vi "dfd_Cascaded SOS Form I Transposed Normalization.vi"(7 "scale type":T1, 9 "coefficients b":dbl[](array[numeric]) format="%.2f", 10 "coefficients a":dbl[](array[numeric]) format="%.2f", 11 "x":dbl[](array[numeric])) -> (2 "norm":dbl[](array[numeric]) format="%.2f", 3 "y":dbl[](array[numeric]))   [LabVIEW 2017, in "NI_DigFilter_FXP.lvlib"]
uses:
  <vilib>/addons/Digital Filter Design/NI_DigFilter_FXP.lvlib
  <vilib>/addons/Digital Filter Design/_Objects.llb/DFD Coef Norm Type.ctl
  <vilib>/addons/Digital Filter Design/NI_DigFilterLicensed.lvlib
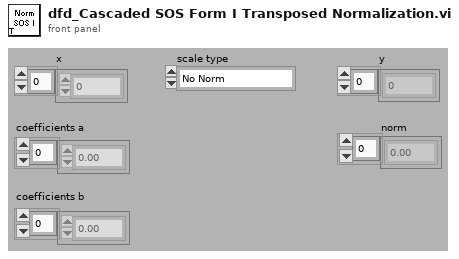
[diagram p1: front panel]
types:
  T1 = typedef "NI_DigFilterLicensed.lvlib/DFD Coef Norm Type.ctl" = enum16{"No Norm", "Time Domain 1-Norm", "Time Domain 2-Norm", "Time Domain Inf-Norm"}
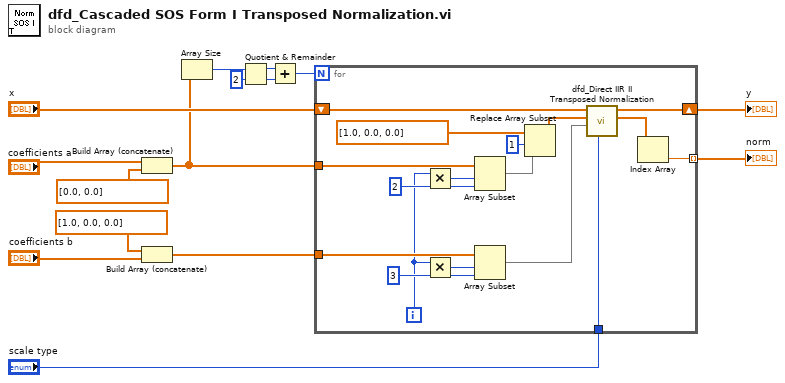
[diagram p0: block diagram]
diagram:
  n1 = Build Array (concatenate)("coefficients a", dbl[] [0.0, 0.0]) -> (w1:dbl[])
  n2 = Build Array (concatenate)(dbl[] [1.0, 0.0, 0.0], "coefficients b") -> (w4:dbl[])
  n3 = Array Size(array=w1) -> (size(s)=w12:i32)
  n4 = Quotient & Remainder(x=w12, y=2) -> (x-y*floor(x/y)=w14:i32, floor(x/y)=w13:i32)
  n5 = Add(x=w14, y=w13) -> (x+y=w11:i32)
  n6 = for {
    N: w11 -> [_]
    tunnel: w4 -> [w32]
    tunnel: w1 -> [w31]
    shift-right: [w17] -> w8
    shift-left: "x" -> [w21]
    tunnel: [w22] -> w7 mode=indexing
    tunnel: "scale type" -> [w20]
    i -> [w26]
    w28 = 2
    w30 = 3
    n7 = Multiply(x=w26, y=w28) -> (x*y=w27:i32)
    n8 = Multiply(x=w26, y=w30) -> (x*y=w29:i32)
    n9 = Array Subset(array=w31, index=w27, length=w28) -> (w24:dbl[])
    n10 = Array Subset(array=w32, index=w29, length=w30) -> (w18:dbl[])
    n11 = Replace Array Subset(array=dbl[] [1.0, 0.0, 0.0], new element=w24, index=1) -> (w19:dbl[])
    n12 = call <vilib>:"dfd_Direct IIR II Transposed Normalization.vi"("scale type"=w20, "coefficients b"=w18, "coefficients a"=w19, "x"=w21) -> ("norm"=w16:dbl[], "y"=w17:dbl[])  [unwired: 6 out]
    n13 = Index Array(array=w16) -> (element=w22:dbl)  [unwired: 1 in]
  }
  "norm" <- w7
  "y" <- w8
